vi "3. Copy Image Symmetry And Merge.vi"() -> ()   [LabVIEW 2019]
doc: "c 2020 ReMiSYS All rights reserved."
uses:
  <vilib>/vision/NI_Vision_Development_Module.lvlib
panel:
  in  "Stop (F)":bool
  out "final":T1(plugin-control)
  out "sym":T1(plugin-control)
  out "ori":T1(plugin-control)
  # "c 2020 ReMiSYS All rights reserved."
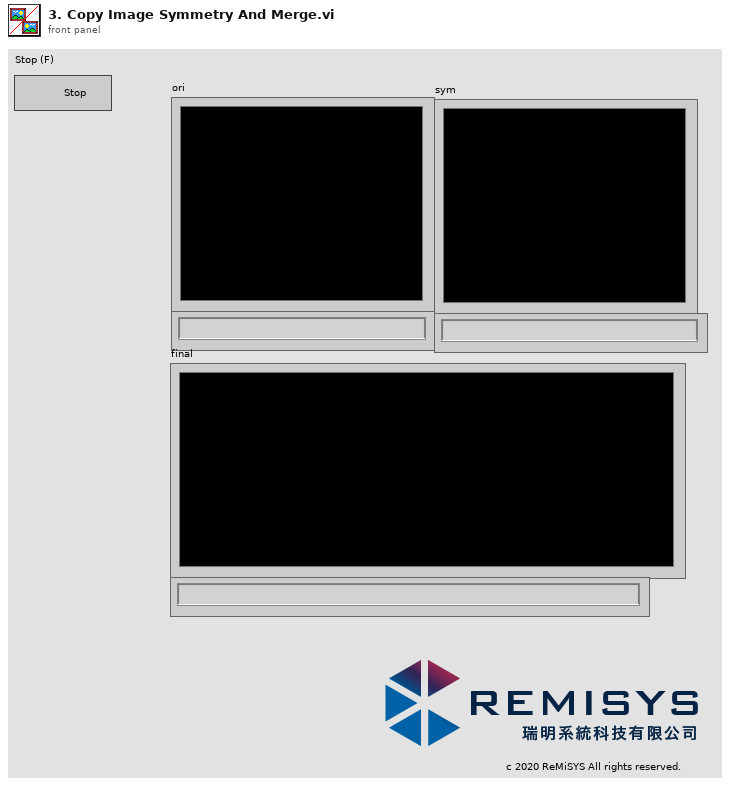
[diagram p1: front panel]
types:
  T1 = typedef "IMAQ Image.ctl" = refnum<image>
  T2 = typedef "Image Type" = u32
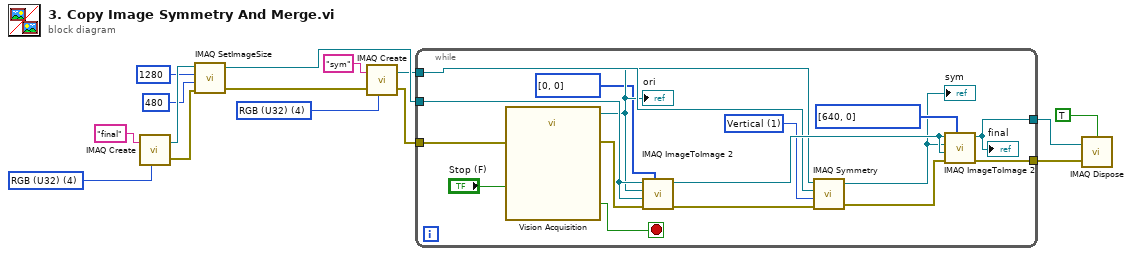
[diagram p0: block diagram]
diagram:
  w5 = T2 4 items=["Grayscale (U8)", "Grayscale (I16)", "Grayscale (SGL)", "Complex (CSG)", "RGB (U32)", "HSL (U32)", "RGB (U64)", "Grayscale (U16)"] ("Image Type")
  w10 = T2 4 items=["Grayscale (U8)", "Grayscale (I16)", "Grayscale (SGL)", "Complex (CSG)", "RGB (U32)", "HSL (U32)", "RGB (U64)", "Grayscale (U16)"] ("Image Type")
  n1 = call "IMAQ Create"("Image Name"="final", "Image Type"=w10) -> ("New Image"=w12:T1, "error out"=w4:errorcluster)  [unwired: 3 in]
  n2 = call "IMAQ SetImageSize"("error in (no error)"=w4, "Y Resolution"=480, "X Resolution"=1280, "Image"=w12) -> ("error out"=w3:errorcluster, "Image Out"=w11:T1)  [unwired: 1 in]
  n3 = call "IMAQ Create"("Image Name"="sym", "Image Type"=w5, "error in (no error)"=w3) -> ("New Image"=w9:T1, "error out"=w2:errorcluster)  [unwired: 2 in]
  n4 = while {
    tunnel: w11 -> [w31]
    tunnel: w9 -> [w24]
    tunnel: [w21] -> w8
    tunnel: w2 -> [w18]
    tunnel: [w16] -> w1
    stop <- w25 stop-if-true
    w27 = u32 1 items=["Horizontal", "Vertical", "Central", "1st Diagonal", "2nd Diagonal"] ("Type of Symmetry")
    n5 = call "Vision Acquisition"("Stop (F)"="Stop (F)", "error in"=w18) -> ("Image Out"=w23:T1, "Stopped"=w25:bool, "error out"=w17:errorcluster)  [unwired: 23 in]
    "ori" <- w23
    n6 = call "IMAQ ImageToImage 2"("Offset Left/Top"=i32[] [0, 0], "error in (no error)"=w17, "Image Dst"=w31, "Image Src (Small)"=w23, "Image Src (Large)"=w31) -> ("error out"=w20:errorcluster, "Image Dst Out"=w30:T1)  [unwired: 5 in]
    n7 = call "IMAQ Symmetry"("error in (no error)"=w20, "Type of Symmetry"=w27, "Image Dst"=w24, "Image Src"=w23) -> ("error out"=w19:errorcluster, "Image Dst Out"=w28:T1)  [unwired: 1 in]
    "sym" <- w28
    n8 = call "IMAQ ImageToImage 2"("Offset Left/Top"=i32[] [640, 0], "error in (no error)"=w19, "Image Dst"=w30, "Image Src (Small)"=w28, "Image Src (Large)"=w30) -> ("error out"=w16:errorcluster, "Image Dst Out"=w21:T1)  [unwired: 5 in]
    "final" <- w21
  }
  n9 = call "IMAQ Dispose"("All Images? (No)"=TRUE, "Image"=w8, "error in (no error)"=w1) -> ()  [unwired: 3 in, 1 out]
